vi "PLC.Dial800.vi"(7 "PLC Indicator":refnum<vi>, 8 "Is Child":bool, 9 "Config Dir":path=path "C:/MTE/Circle Test/Config", 10 "Name":string="PLC", 11 "TE Q":refnum<queue>) -> ()   [LabVIEW 2018]
uses:
  SubVIs/PLC.800 Variables.ctl
  <vilib>/KATE/Queues/Q.Element.ctl
  SubVIs/PLC.Dial800.Var URL Item.ctl
  SubVIs/PLC.Dial800.VarNameSelector.ctl
  SubVIs/PLC.Dial800.OPC Server Config.ctl
  SubVIs/PLC.Dial800.VarNames.ctl
  Beckhoff/Dial 750/Controls/PLC750.Connection Config.ctl
  <vilib>/KATE/Queues/Queue Utils.lvlib
  <vilib>/KATE/Scheduler/Scheduler.lvlib
  <vilib>/KATE/Status/Status Utils.lvlib
panel:
  out "Nest":i32
  out "Test State 2":T1(radio)
  out "Connected":bool
  in  "Tab Control":enum32{"Operate", "Config", "Maint"}(tab)
  out "PLC HB Err Msg":string="PLC Hearbeat Error"
  out "PLC HB Err":bool
  in  "SN Set":bool
  in  "SN Input":string caption="SN"
  in  "Reset Clear":bool
  in  "Reset Set":bool
  in  "Run Clear":bool
  in  "Run Set":bool
  in  "Start Clear":bool
  in  "Seq Done FAIL":bool
  in  "Seq Run":bool
  in  "Seq Done PASS":bool
  out "Status":string
  out "SN":string
  out "Test State":T1(radio)
  out "Reading":bool
  out "PLC Variables":T2
  in  "Start Set":bool
  out "Test Running":bool
  out "Result":string
  out "Read Time":timestamp format="%<%.3X>T"
  in  "PLC Read Interval(s)":dbl=0.1 caption="Read Interval(s)" format="%#_13g"
  in  "Read Data":bool
  out "ReadDur(s)":dbl format="%.3f"
  in  "Reset":bool
  out "OPC Server":T3={"IP"="localhost", "Topic"="Stn800", "Server"="RSLinx OPC Server", "VarRoot"="Program:Stn001_90_OffloadMain", "TestPCArray"="TestPC", "VarNames"={"SN"="SN", "Reset"="Reset", "HeartbeatPLC"="HeartbeatPLC", "HeartbeatPC"="HeartbeatTestPC", "Start"="Start", "Running"="Running", "Done"="Done", "Pass"="Pass"}}
  out "Var URLs":T5[](array[typedef])
  in  "PLC HB TimeOut(s)":dbl=5.0 caption="PLC Heartbeat Timeout(s)" format="%#_13g"
  in  "Retry Sec":dbl=2.0 caption="Connect Retry Sec" format="%#_13g"
  out "Error":errorcluster
  in  "Clear Error":bool
  out "Error Time":timestamp format="%<%.3X>T"
  in  "Exit":bool
  in  "Simulate":bool
  in  "Single Step":bool
  in  "Enabled":bool=TRUE
  # "PLC Connection Manager"
  # "Manual Ctrl"
  # "Test Executive Data"
  # "Start"
  # "Running"
  # "Result\nDone"
  # "Simulate TE"
  # "Reset"
  # "(Access path)"
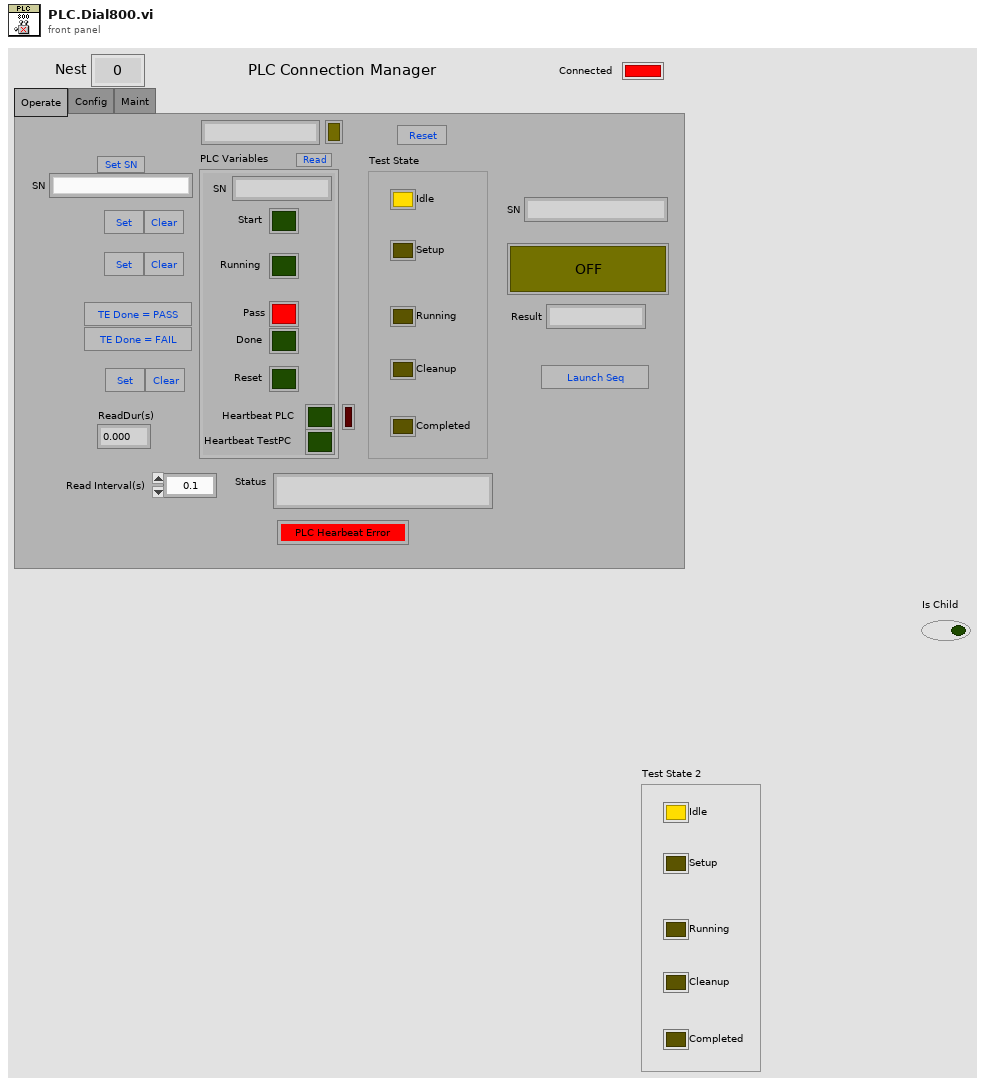
[diagram p1: front panel]
types:
  T1 = enum32{"Idle", "Setup", "Running", "Cleanup", "Completed"}
  T2 = typedef "PLC.800 Variables.ctl" = cluster{"SN":string, "Start":bool, "Pass":bool, "Done":bool, "Running":bool, "Heartbeat PLC":bool, "Heartbeat TestPC":bool, "Reset":bool}
  T3 = typedef "PLC.Dial800.OPC Server Config.ctl" = cluster{"IP":string, "Topic":string, "Server":string, "VarRoot":string, "TestPCArray":string, "VarNames":T4}
  T4 = typedef "PLC.Dial800.VarNames.ctl" = cluster{"SN":string, "Reset":string, "HeartbeatPLC":string, "HeartbeatPC":string, "Start":string, "Running":string, "Done":string, "Pass":string}
  T5 = typedef "PLC.Dial800.Var URL Item.ctl" = cluster{"Var":T6, "URL":string, "Socket ID":refnum<k13>}
  T6 = typedef "PLC.Dial800.VarNameSelector.ctl" = enum16{"SN", "Reset", "HeartBeat_PLC", "Heartbeat_PC", "Start", "Running", "Done", "Pass"}
  T7 = enum32{"invalid app kind", "Development System", "Run Time System", "Student Edition", "Embedded LabVIEW", "Evaluation", "Custom"}
  T8 = enum8{"Enabled", "Disabled", "Disabled and Grayed Out"}
  T9 = enum32{"Invalid", "Standard", "Closed", "Hidden", "Minimized", "Maximized"}
  T10 = typedef "PLC750.Connection Config.ctl" = cluster{"Net ID Target":string, "Net ID Source":string, "IP Address Target":string, "Target Port":u16}
  T11 = cluster{"OPC Server":T3, "Var URLs":T5[], "Data":T2, "Nest":i32, "Connected":bool, "ConCfg":T10, "State":enum32{"Idle", "Setup", "Running", "Cleanup", "Completed"}, "PLC Indicator":refnum<vi>, "HeartBeat":bool, "TE Running":bool, "Cleanup":bool, "Reset":bool, "HB PLC Trans":timestamp, "HB PLC Last State":bool, "PLC HB Err":bool}
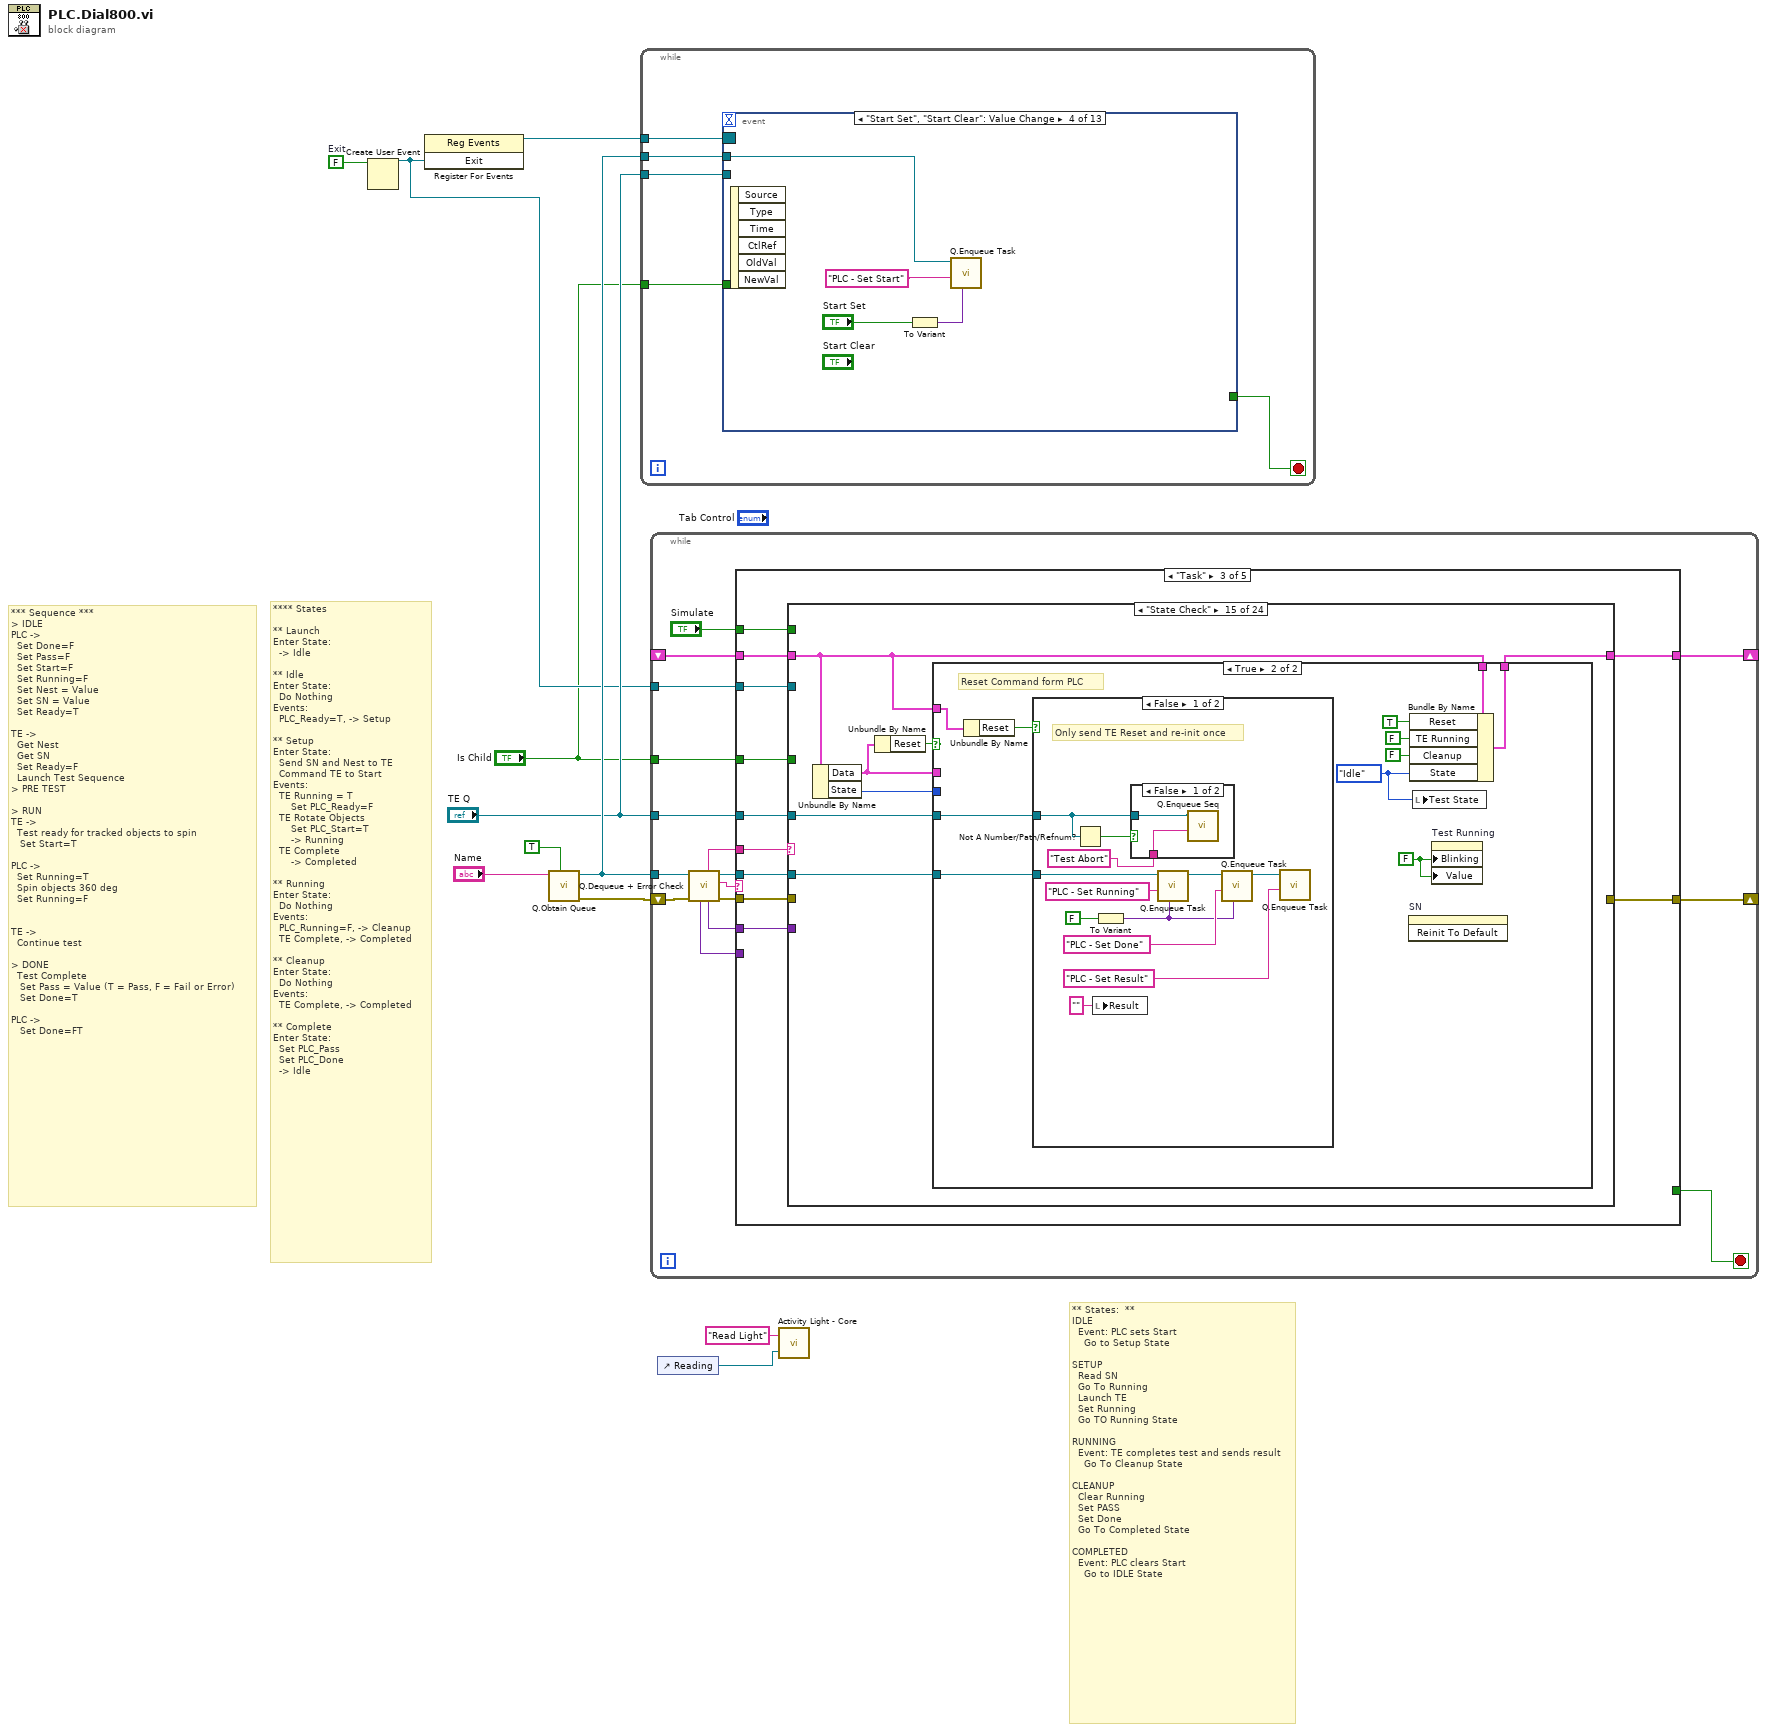
[diagram p0: block diagram]
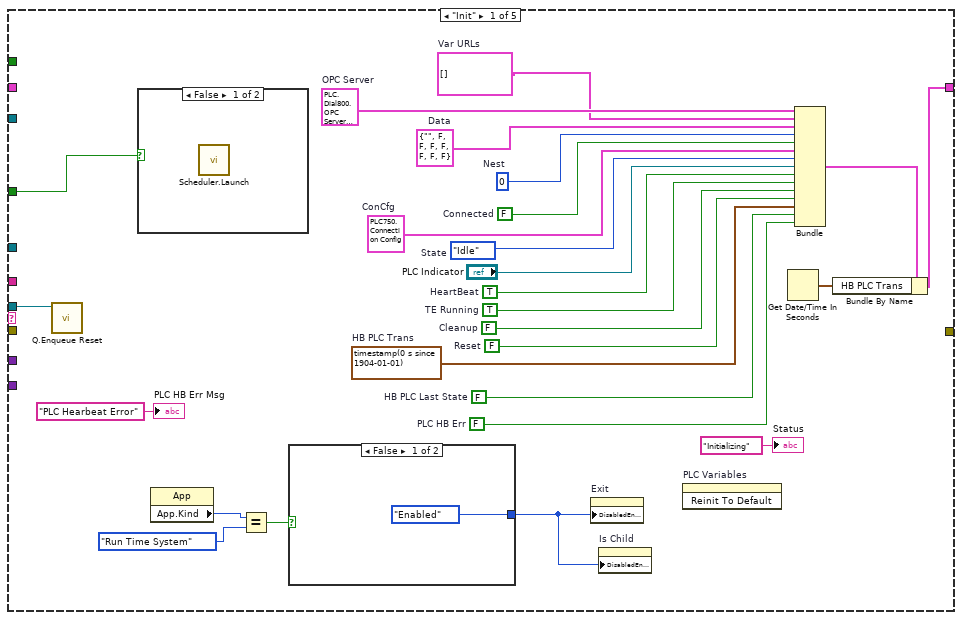
[diagram p2: hidden frame]
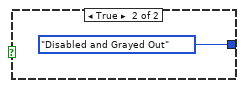
[diagram p3: hidden frame]
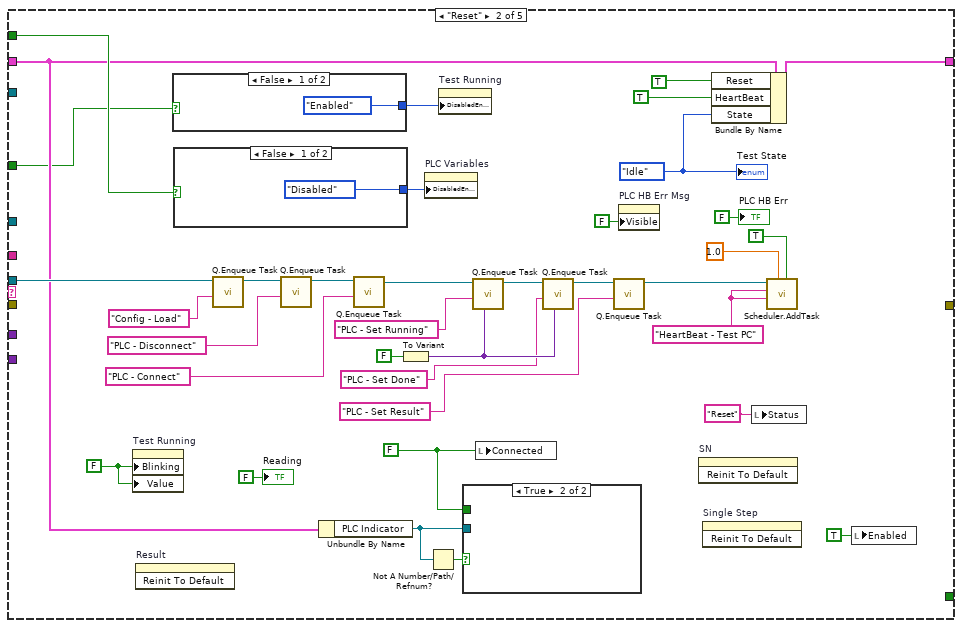
[diagram p5: hidden frame]
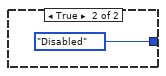
[diagram p6: hidden frame]
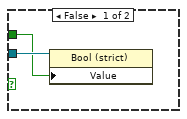
[diagram p7: hidden frame]
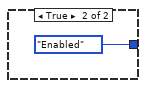
[diagram p8: hidden frame]
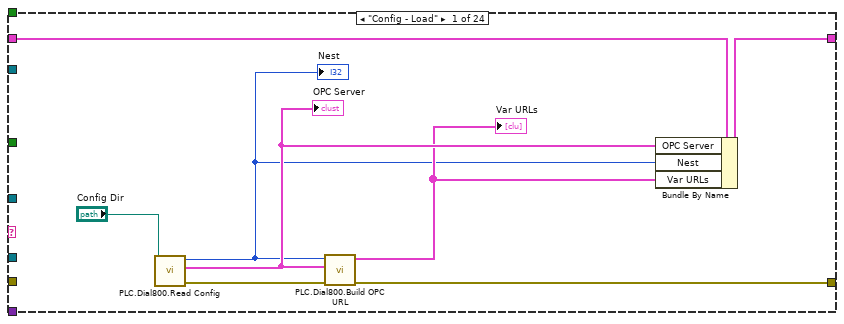
[diagram p9: hidden frame]
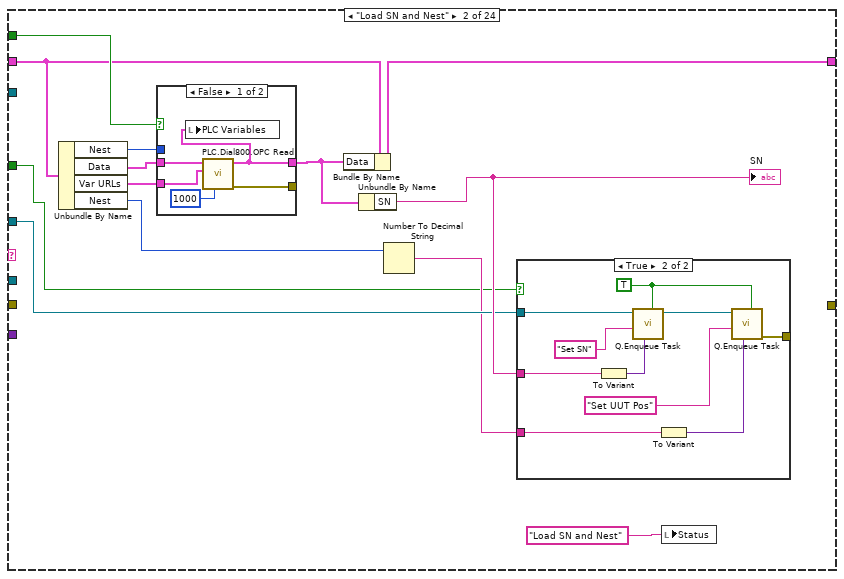
[diagram p10: hidden frame]
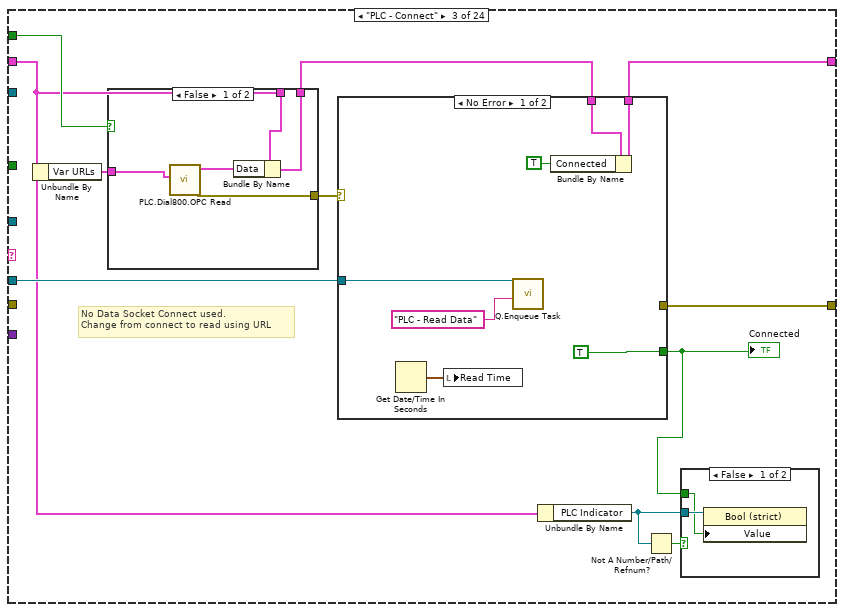
[diagram p13: hidden frame]
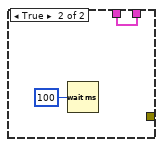
[diagram p15: hidden frame]
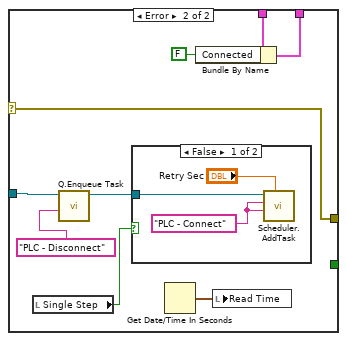
[diagram p16: hidden frame]
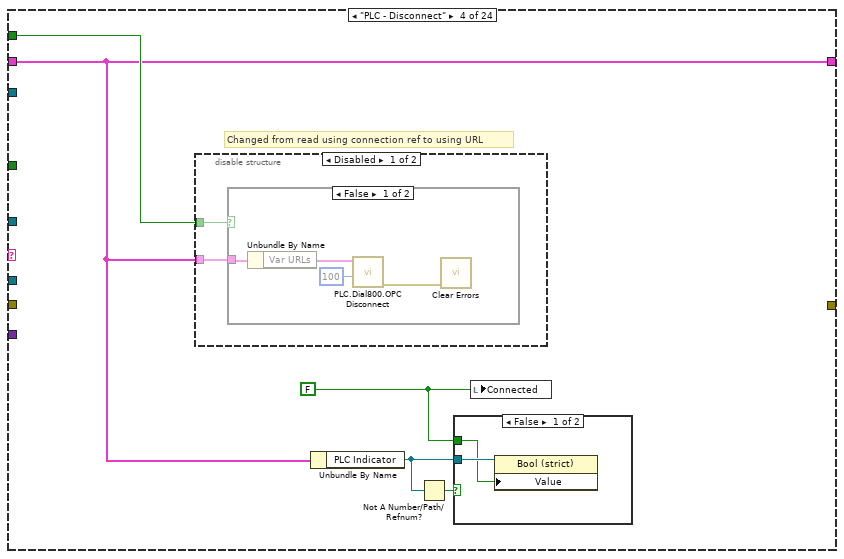
[diagram p18: hidden frame]
diagram:
  w8 = FALSE  # Exit
  # "** States:  ** \nIDLE\n  Event: PLC sets Start\n    Go to Setup State\n\nSETUP\n  Read SN\n  Go To Running\n  Launch TE\n  Set Running\n  Go TO Running State\n\nRUNNING\n  Event: TE completes test and sends result\n    Go To Cleanup State\n\nCLEANUP\n  Clear Running\n  Set PASS\n  Set Done\n  Go To Completed State\n\nCOMPLETED\n  Event: PLC clears Start\n    Go to IDLE State"
  # "**** States\n\n** Launch\nEnter State: \n  -> Idle\n\n** Idle\nEnter State: \n  Do Nothing\nEvents:\n  PLC_Ready=T, -> Setup\n\n** Setup\nEnter State: \n  Send SN and Nest to TE\n  Command TE to Start\nEvents:\n  TE Running = T\n      Set PLC_Ready=F\n  TE Rotate Objects\n      Set PLC_Start=T\n      -> Running\n  TE Complete\n      -> Completed\n\n** Running\nEnter State: \n  Do Nothing\nEvents:\n  PLC_Running=F, -> Cleanup\n  TE Complete, -> Completed\n\n** Cleanup\nEnter State: \n  Do Nothing\nEvents:\n  TE Complete, -> Completed\n\n** Complete\nEnter State: \n  Set PLC_Pass\n  Set PLC_Done \n  -> Idle"
  # "*** Sequence ***\n> IDLE\nPLC -> \n  Set Done=F\n  Set Pass=F\n  Set Start=F\n  Set Running=F\n  Set Nest = Value\n  Set SN = Value\n  Set Ready=T\n\nTE -> \n  Get Nest\n  Get SN\n  Set Ready=F\n  Launch Test Sequence\n> PRE TEST\n  \n> RUN\nTE -> \n  Test ready for tracked objects to spin\n   Set Start=T\n\nPLC -> \n  Set Running=T\n  Spin objects 360 deg\n  Set Running=F\n\n\nTE -> \n  Continue test\n\n> DONE\n  Test Complete\n   Set Pass = Value (T = Pass, F = Fail or Error)\n   Set Done=T\n\nPLC -> \n   Set Done=FT"
  n1 = Create User Event(user event datatype=w8) -> (user event=w4:refnum<user-event>)  [unwired: 1 in, 1 out]
  n2 = register-events(w4) -> (reference out=w7:refnum<event-registration>)  [unwired: 2 in, 1 out]
  n3 = call <vilib>:"Q.Obtain Queue.vi"("Enqueue Init"=TRUE, "Q Name"="Name") -> ("error out"=w5:errorcluster, "Q Out"=w9:refnum<queue>)  [unwired: 7 in, 1 out]
  n4 = while {
    tunnel: w9 -> [w16]
    tunnel: w7 -> [w15]
    tunnel: "TE Q" -> [w14]
    tunnel: "Is Child" -> [w12]
    stop <- w13 stop-if-true
    n5 = event shown="[3] \"Start Set\", \"Start Clear\": Value Change" {
      selector: w15 -> [_ _ _ _ _ _ _ _ _ _ _ _ _]
      dyn-events: _ -> [_ _ _ _ _ _ _ _ _ _ _ _ _]
      timeout: _ -> [_ _ _ _ _ _ _ _ _ _ _ _ _]
      tunnel: w16 -> [_ w17 w18 w23 w27 w31 w33 w39 w45 _ w49 w55 w56]
      tunnel: w14 -> [_ _ _ _ _ _ _ _ _ _ _ _ _]
      tunnel: [_ _ _ _ _ _ _ _ _ TRUE w48 TRUE _] -> w13
      tunnel: w12 -> [_ _ _ _ _ _ _ _ _ _ w47 _ _]
      event "Clear Error": Value Change {
        n6 = event-data() -> ()  [unwired: 1 in, 6 out]
        n7 = invoke on="Error" class="Clust (strict)" method="Reinit To Default"() -> ()  [unwired: 3 in, 3 out]
      }
      event "Reset": Value Change {
        n8 = event-data() -> ()  [unwired: 1 in, 6 out]
        n9 = call <vilib>:"Q.Enqueue Reset.vi"("Q In"=w17) -> ()  [unwired: 9 in, 2 out]
      }
      event "Read Data": Value Change {
        n10 = event-data() -> ()  [unwired: 1 in, 6 out]
        n11 = call <vilib>:"Q.Enqueue Task.vi"("Task Name"="PLC - Read Data", "Q In"=w18) -> ()  [unwired: 8 in, 2 out]
      }
      event "Start Set", "Start Clear": Value Change {
        n12 = event-data() -> ()  [unwired: 1 in, 6 out]
        n13 = To Variant(anything="Start Set") -> (Variant=w21:variant)
        n14 = call <vilib>:"Q.Enqueue Task.vi"("Data1"=w21, "Task Name"="PLC - Set Start", "Q In"=w23) -> ()  [unwired: 7 in, 2 out]
      }
      event "Run Set", "Run Clear": Value Change {
        n15 = event-data() -> ()  [unwired: 1 in, 6 out]
        n16 = To Variant(anything="Run Set") -> (Variant=w25:variant)
        n17 = call <vilib>:"Q.Enqueue Task.vi"("Data1"=w25, "Task Name"="PLC - Set Running", "Q In"=w27) -> ()  [unwired: 7 in, 2 out]
      }
      event "Reset Set", "Reset Clear": Value Change {
        n18 = event-data() -> ()  [unwired: 1 in, 6 out]
        n19 = To Variant(anything="Reset Set") -> (Variant=w29:variant)
        n20 = call <vilib>:"Q.Enqueue Task.vi"("Data1"=w29, "Task Name"="PLC - Set Reset", "Q In"=w31) -> ()  [unwired: 7 in, 2 out]
      }
      event "SN Set": Value Change {
        n21 = event-data() -> ()  [unwired: 1 in, 6 out]
        n22 = call <vilib>:"Q.Enqueue Task.vi"("Task Name"="PLC - Set SN", "Q In"=w33) -> ()  [unwired: 8 in, 2 out]
      }
      event "Seq Done PASS": Value Change {
        n23 = event-data() -> ()  [unwired: 1 in, 6 out]
        n24 = To Variant(anything="PASS") -> (Variant=w34:variant)
        n25 = call <vilib>:"Q.Enqueue Task.vi"("Data1"=w34, "Task Name"="TE Result", "Q In"=w39) -> ("Q Out"=w37:refnum<queue>)  [unwired: 7 in, 1 out]
        n26 = call <vilib>:"Q.Enqueue Task.vi"("Task Name"="TE Complete", "Q In"=w37) -> ()  [unwired: 8 in, 2 out]
      }
      event "Seq Done FAIL": Value Change {
        n27 = event-data() -> ()  [unwired: 1 in, 6 out]
        n28 = To Variant(anything="FAIL") -> (Variant=w40:variant)
        n29 = call <vilib>:"Q.Enqueue Task.vi"("Data1"=w40, "Task Name"="TE Result", "Q In"=w45) -> ("Q Out"=w43:refnum<queue>)  [unwired: 7 in, 1 out]
        n30 = call <vilib>:"Q.Enqueue Task.vi"("Task Name"="TE Complete", "Q In"=w43) -> ()  [unwired: 8 in, 2 out]
      }
      event User Event {
        n31 = event-data() -> ()  [unwired: 1 in, 4 out]
      }
      event Panel Close? {
        n32 = event-data() -> ()  [unwired: 1 in, 4 out]
        n33 = case shown="False" w47 {
          tunnel: w49 -> [w52 _]
          tunnel: [TRUE _] -> w48
          frame False {
            n34 = call <vilib>:"Q.Enqueue Exit.vi"("Q In"=w52) -> ()  [unwired: 9 in, 2 out]
          }
          frame True {
            n35 = control-ref of="This VI"() -> (w53:refnum<vi>)
            n36 = invoke class="VI" method="FP.Close"(reference=w53) -> ()  [unwired: 2 in, 3 out]
          }
        }
        n37 = event-data("Discard?"=TRUE) -> ()  [unwired: 1 in, 1 out]
      }
      event "Exit": Value Change {
        n38 = event-data() -> ()  [unwired: 1 in, 6 out]
        n39 = call <vilib>:"Q.Enqueue Exit.vi"("Q In"=w55) -> ()  [unwired: 9 in, 2 out]
      }
      event "Seq Run": Value Change {
        n40 = event-data() -> ()  [unwired: 1 in, 6 out]
        n41 = call <vilib>:"Q.Enqueue Task.vi"("Task Name"="TE Running", "Q In"=w56) -> ()  [unwired: 8 in, 2 out]
      }
    }
  }
  n42 = while {
    tunnel: w9 -> [w73]
    shift-right: [w65] -> _
    shift-left: _ -> [w72]
    tunnel: "TE Q" -> [w63]
    shift-right: [w61] -> _
    shift-left: w5 -> [w62]
    tunnel: w4 -> [w60]
    tunnel: "Is Child" -> [w58]
    stop <- w64 stop-if-true
    n43 = call <vilib>:"Q.Dequeue + Error Check.vi"("Error In"=w62, "Q In"=w73) -> ("error out"=w69:errorcluster, "Cmd"=w71:string, "Q Out"=w70:refnum<queue>, "Data1"=w67:variant, "Sub"=w68:string, "Data2"=w66:variant)  [unwired: 4 in]
    n44 = case shown="\"Task\"" w71 {
      tunnel: w72 -> [_ w122 w150 w715 w726]
      tunnel: w70 -> [w96 w132 w152 _ w725]
      tunnel: w69 -> [_ _ w151 w718 _]
      tunnel: w68 -> [_ _ w154 w719 _]
      tunnel: w67 -> [_ _ w153 w716 _]
      tunnel: w66 -> [_ _ _ _ _]
      tunnel: [w75 w133 w149 w715 w726] -> w65
      tunnel: [_ _ _ _ TRUE] -> w64
      tunnel: w63 -> [_ _ w145 _ _]
      tunnel: [_ _ w148 _ _] -> w61
      tunnel: w60 -> [_ _ w147 _ w733]
      tunnel: "Simulate" -> [_ w128 w146 _ w727]
      tunnel: w58 -> [w92 w120 w144 _ w731]
      frame "Init" {
        w77 = FALSE  # PLC HB Err
        w79 = FALSE  # HB PLC Last State
        w80 = timestamp(0 s since 1904-01-01)  # HB PLC Trans
        w81 = FALSE  # Reset
        w82 = FALSE  # Cleanup
        w83 = TRUE  # TE Running
        w84 = TRUE  # HeartBeat
        w85 = T2 {"SN"="", "Start"=FALSE, "Pass"=FALSE, "Done"=FALSE, "Running"=FALSE, "Heartbeat PLC"=FALSE, "Heartbeat TestPC"=FALSE, "Reset"=FALSE}  # Data
        w86 = T5[] []  # Var URLs
        w87 = T3 {"IP"="localhost", "Topic"="Stn800", "Server"="RSLinx OPC Server", "VarRoot"="Program:Stn001_90_OffloadMain", "TestPCArray"="TestPC", "VarNames"={"SN"="SN", "Reset"="Reset", "HeartbeatPLC"="HeartbeatPLC", "HeartbeatPC"="HeartbeatTestPC", "Start"="Start", "Running"="Running", "Done"="Done", "Pass"="Pass"}}  # OPC Server
        w95 = T1."Idle"  # State
        w97 = T10 {"Net ID Target"="5.49.203.74.1.1", "Net ID Source"="192.168.1.18.1.1", "IP Address Target"="172.16.113.5", "Target Port"=851}  # ConCfg
        w98 = FALSE  # Connected
        w99 = 0  # Nest
        n45 = call <vilib>:"Q.Enqueue Reset.vi"("Q In"=w96) -> ()  [unwired: 9 in, 2 out]
        n46 = case shown="False" w92 {
          frame False {
            n47 = call <vilib>:"Scheduler.Launch.vi"() -> ()  [unwired: 9 in, 3 out]
          }
          frame True {
          }
        }
        n48 = property class="App"() -> ("App.Kind"=w90:T7)  [unwired: 2 in, 2 out]
        n49 = Equal?(x=w90, y=T7."Run Time System" ("Application:Kind")) -> (x = y?=w88:bool)
        n50 = case shown="False" w88 {
          tunnel: [T8."Enabled" ("Disabled") T8."Disabled and Grayed Out" ("Disabled")] -> w91
          frame False {
          }
          frame True {
          }
        }
        n51 = property on="Exit" class="Bool"("DisabledEnum"=w91) -> ()  [unwired: 2 in, 2 out]
        n52 = property on="Is Child" class="Bool (strict)"("DisabledEnum"=w91) -> ()  [unwired: 2 in, 2 out]
        n53 = invoke on="PLC Variables" class="Clust (strict)" method="Reinit To Default"() -> ()  [unwired: 3 in, 3 out]
        n54 = Get Date/Time In Seconds() -> (seconds since 1Jan1904=w74:timestamp)
        n55 = Bundle("OPC Server"=w87, "Var URLs"=w86, "Data"=w85, "Nest"=w99, "Connected"=w98, "ConCfg"=w97, "State"=w95, "PLC Indicator"="PLC Indicator", "HeartBeat"=w84, "TE Running"=w83, "Cleanup"=w82, "Reset"=w81, "HB PLC Trans"=w80, "HB PLC Last State"=w79, "PLC HB Err"=w77) -> (w76:T11)  [unwired: 1 in]
        n56 = Bundle By Name(cluster=w76, "HB PLC Trans"=w74) -> (w75:T11)
        "Status" <- "Initializing" ("Activity")
        "PLC HB Err Msg" <- "PLC Hearbeat Error" ("PLC HB Err Msg")
      }
      frame "Reset" {
        w117 = "HeartBeat - Test PC" ("Sched Name")
        w129 = T1."Idle" ("Test State")
        w123 = FALSE ("Connected")
        w131 = FALSE ("Blinking")
        n57 = property on="Test Running" class="Bool (strict)"("Blinking"=w131, "Value"=w131) -> ()  [unwired: 2 in, 2 out]
        n58 = invoke on="Result" class="Str" method="Reinit To Default"() -> ()  [unwired: 3 in, 3 out]
        n59 = case shown="False" w120 {
          tunnel: [T8."Enabled" ("Disabled") T8."Disabled" ("Disabled")] -> w121
          frame False {
          }
          frame True {
          }
        }
        n60 = case shown="False" w128 {
          tunnel: [T8."Disabled" ("Disabled") T8."Enabled" ("Disabled")] -> w127
          frame False {
          }
          frame True {
          }
        }
        n61 = call <vilib>:"Q.Enqueue Task.vi"("Task Name"="Config - Load", "Q In"=w132) -> ("Q Out"=w134:refnum<queue>)  [unwired: 8 in, 1 out]
        n62 = call <vilib>:"Q.Enqueue Task.vi"("Task Name"="PLC - Disconnect", "Q In"=w134) -> ("Q Out"=w113:refnum<queue>)  [unwired: 8 in, 1 out]
        n63 = Unbundle By Name(w122) -> ("PLC Indicator"=w124:refnum<vi>)
        n64 = call <vilib>:"Q.Enqueue Task.vi"("Task Name"="PLC - Connect", "Q In"=w113) -> ("Q Out"=w105:refnum<queue>)  [unwired: 8 in, 1 out]
        n65 = To Variant(anything=FALSE) -> (Variant=w111:variant)
        n66 = property on="PLC Variables" class="Clust (strict)"("DisabledEnum"=w127) -> ()  [unwired: 2 in, 2 out]
        n67 = Not A Number/Path/Refnum?(number/path/refnum=w124) -> (NaN/Path/Refnum?=w125:bool)
        n68 = property on="Test Running" class="Bool (strict)"("DisabledEnum"=w121) -> ()  [unwired: 2 in, 2 out]
        n69 = case shown="True" w125 {
          tunnel: w124 -> [w141 _]
          tunnel: w123 -> [w140 _]
          frame False {
            n70 = property class="Bool (strict)"(reference=w141, "Value"=w140) -> ()  [unwired: 1 in, 2 out]
          }
          frame True {
          }
        }
        n71 = call <vilib>:"Q.Enqueue Task.vi"("Data1"=w111, "Task Name"="PLC - Set Running", "Q In"=w105) -> ("Q Out"=w110:refnum<queue>)  [unwired: 7 in, 1 out]
        n72 = local write "Connected"(w123) -> ()
        n73 = call <vilib>:"Q.Enqueue Task.vi"("Data1"=w111, "Task Name"="PLC - Set Done", "Q In"=w110) -> ("Q Out"=w112:refnum<queue>)  [unwired: 7 in, 1 out]
        n74 = call <vilib>:"Q.Enqueue Task.vi"("Task Name"="PLC - Set Result", "Q In"=w112) -> ("Q Out"=w104:refnum<queue>)  [unwired: 8 in, 1 out]
        n75 = property on="PLC HB Err Msg" class="Str"("Visible"=FALSE) -> ()  [unwired: 2 in, 2 out]
        n76 = invoke on="SN" class="Str" method="Reinit To Default"() -> ()  [unwired: 3 in, 3 out]
        n77 = invoke on="Single Step" class="Bool (strict)" method="Reinit To Default"() -> ()  [unwired: 3 in, 3 out]
        n78 = Bundle By Name(cluster=w122, "Reset"=TRUE ("HeartBeat"), "HeartBeat"=TRUE, "State"=w129) -> (w133:T11)
        n79 = local write "Status"("Reset" ("Activity")) -> ()
        n80 = call <vilib>:"Scheduler.AddTask.vi"("Recurring"=TRUE, "Interval(s)"=1.0, "Task Name"=w117, "Sched Name"=w117, "Q In"=w104) -> ()  [unwired: 5 in, 2 out]
        n81 = local write "Enabled"(TRUE ("Enabled")) -> ()
        "Reading" <- FALSE ("Reading")
        "Test State" <- w129
        "PLC HB Err" <- FALSE ("PLC HB Err")
      }
      frame "Task" {
        n82 = case shown="\"State Check\"" w154 {
          tunnel: w153 -> [_ _ _ _ _ w284 w311 w338 w365 _ _ _ _ _ _ _ _ w667 _ _ _ w703 _ _]
          tunnel: w152 -> [_ _ w200 _ w256 _ _ _ _ _ _ w443 w473 w502 w532 _ w660 _ _ w671 w674 w700 w710 _]
          tunnel: w151 -> [_ _ _ _ w244 _ _ _ _ _ _ _ _ _ _ _ _ _ _ _ _ _ _ _]
          tunnel: w150 -> [w160 w164 w193 w232 w255 w281 w308 w335 w362 w390 w419 w446 w479 w500 w528 w652 w663 w668 w669 w670 w677 w698 w705 w713]
          tunnel: [w161 w167 w201 w232 w254 w281 w308 w335 w362 w390 w419 w449 w478 w499 w531 w652 w662 w668 w669 w670 w676 w697 w704 w713] -> w149
          tunnel: [w157 _ w199 _ w251 w287 w314 w341 w368 w393 w423 w451 _ _ _ _ _ _ _ _ _ _ _ _] -> w148
          tunnel: w147 -> [_ _ _ _ _ _ _ _ _ _ _ _ _ _ _ _ _ _ _ _ _ _ _ _]
          tunnel: w146 -> [_ w165 w197 w235 w249 w285 w312 w339 w366 w391 w420 w453 _ _ _ _ _ _ _ _ w673 _ _ _]
          tunnel: w145 -> [_ w173 _ _ _ _ _ _ _ _ _ _ _ w503 w530 _ _ _ _ _ w679 _ _ _]
          tunnel: w144 -> [_ w171 _ _ _ _ _ _ _ _ _ _ _ _ _ _ _ _ _ _ w678 _ _ _]
          frame "Config - Load" {
            n83 = call "PLC.Dial800.Read Config.vi"("Config Folder"="Config Dir") -> ("error out"=w158:errorcluster, "OPC Server"=w159:T3, "Nest"=w155:i32)  [unwired: 8 in]
            "OPC Server" <- w159
            "Nest" <- w155
            n84 = call "PLC.Dial800.Build OPC URL.vi"("error in (no error)"=w158, "OPC Server"=w159, "Nest"=w155) -> ("error out"=w157:errorcluster, "Var URLs"=w156:T5[])  [unwired: 7 in]
            "Var URLs" <- w156
            n85 = Bundle By Name(cluster=w160, "OPC Server"=w159, "Nest"=w155, "Var URLs"=w156) -> (w161:T11)
          }
          frame "Load SN and Nest" {
            n86 = Unbundle By Name(w164) -> ("Nest"=w168:i32, "Data"=w169:T2, "Var URLs"=w170:T5[], "Nest"=w163:i32)
            n87 = case shown="False" w165 {
              tunnel: w168 -> [_ _]
              tunnel: w169 -> [w180 w181]
              tunnel: w170 -> [w179 _]
              tunnel: [w176 w181] -> w166
              tunnel: [w178 _] -> _
              frame False {
                n88 = call "PLC.Dial800.OPC Read.vi"("Timeout_ms"=1000, "Var URLs"=w179, "PLC Variables In"=w180) -> ("error out"=w178:errorcluster, "PLC Variables"=w176:T2)  [unwired: 6 in, 1 out]
                n89 = local write "PLC Variables"(w176) -> ()
              }
              frame True {
              }
            }
            n90 = Bundle By Name(cluster=w164, "Data"=w166) -> (w167:T11)
            n91 = Unbundle By Name(w166) -> ("SN"=w174:string)
            "SN" <- w174
            n92 = Number To Decimal String(number=w163) -> (decimal integer string=w172:string)  [unwired: 1 in]
            n93 = case shown="True" w171 {
              tunnel: w174 -> [_ w191]
              tunnel: w173 -> [_ w190]
              tunnel: w172 -> [_ w189]
              tunnel: [_ w183] -> _
              frame False {
              }
              frame True {
                w182 = TRUE ("Top of Q")
                n94 = To Variant(anything=w191) -> (Variant=w188:variant)
                n95 = call <vilib>:"Q.Enqueue Task.vi"("Top of Q"=w182, "Data1"=w188, "Task Name"="Set SN", "Q In"=w190) -> ("Q Out"=w184:refnum<queue>)  [unwired: 6 in, 1 out]
                n96 = To Variant(anything=w189) -> (Variant=w186:variant)
                n97 = call <vilib>:"Q.Enqueue Task.vi"("Top of Q"=w182, "Data1"=w186, "Task Name"="Set UUT Pos", "Q In"=w184) -> ("error out"=w183:errorcluster)  [unwired: 6 in, 1 out]
              }
            }
            n98 = local write "Status"("Load SN and Nest" ("Activity")) -> ()
          }
          frame "PLC - Connect" {
            # "No Data Socket Connect used.\nChange from connect to read using URL"
            n99 = Unbundle By Name(w193) -> ("Var URLs"=w198:T5[])
            n100 = case shown="False" w197 {
              tunnel: [w205 _] -> w202
              tunnel: w198 -> [w207 _]
              tunnel: w193 -> [w209 w210]
              tunnel: [w208 w210] -> w192
              frame False {
                n101 = call "PLC.Dial800.OPC Read.vi"("Var URLs"=w207) -> ("error out"=w205:errorcluster, "PLC Variables"=w206:T2)  [unwired: 8 in, 1 out]
                n102 = Bundle By Name(cluster=w209, "Data"=w206) -> (w208:T11)
              }
              frame True {
                n103 = Wait (ms)(milliseconds to wait=u32 100) -> ()  [unwired: 1 out]
              }
            }
            n104 = case shown="No Error" w202 {
              selector: w202 -> [_ w224]
              tunnel: [w218 w226] -> w201
              tunnel: w192 -> [w217 w227]
              tunnel: w200 -> [w214 w221]
              tunnel: [TRUE _] -> w194
              tunnel: [_ w224] -> w199
              frame No Error {
                n105 = Get Date/Time In Seconds() -> (seconds since 1Jan1904=w212:timestamp)
                n106 = local write "Read Time"(w212) -> ()
                n107 = call <vilib>:"Q.Enqueue Task.vi"("Task Name"="PLC - Read Data" ("Sched Name"), "Q In"=w214) -> ()  [unwired: 8 in, 2 out]
                n108 = Bundle By Name(cluster=w217, "Connected"=TRUE) -> (w218:T11)
              }
              frame Error {
                n109 = local read "Single Step"() -> (w223:bool)
                n110 = call <vilib>:"Q.Enqueue Task.vi"("Task Name"="PLC - Disconnect" ("Sched Name"), "Q In"=w221) -> ("Q Out"=w220:refnum<queue>)  [unwired: 8 in, 1 out]
                n111 = case shown="False" w223 {
                  tunnel: w220 -> [w228 _]
                  frame False {
                    w230 = "PLC - Connect" ("Sched Name")
                    n112 = call <vilib>:"Scheduler.AddTask.vi"("Interval(s)"="Retry Sec", "Task Name"=w230, "Sched Name"=w230, "Q In"=w228) -> ()  [unwired: 6 in, 2 out]
                  }
                  frame True {
                  }
                }
                n113 = Get Date/Time In Seconds() -> (seconds since 1Jan1904=w222:timestamp)
                n114 = Bundle By Name(cluster=w227, "Connected"=FALSE) -> (w226:T11)
                n115 = local write "Read Time"(w222) -> ()
              }
            }
            "Connected" <- w194
            n116 = Unbundle By Name(w193) -> ("PLC Indicator"=w195:refnum<vi>)
            n117 = Not A Number/Path/Refnum?(number/path/refnum=w195) -> (NaN/Path/Refnum?=w196:bool)
            n118 = case shown="False" w196 {
              tunnel: w195 -> [w204 _]
              tunnel: w194 -> [w203 _]
              frame False {
                n119 = property class="Bool (strict)"(reference=w204, "Value"=w203) -> ()  [unwired: 1 in, 2 out]
              }
              frame True {
              }
            }
          }
          frame "PLC - Disconnect" {
            w231 = FALSE ("Connected")
            # "Changed from read using connection ref to using URL"
            n120 = disable-structure shown="Disabled" {
              disable-tunnel: w235 -> [w237 _]
              disable-tunnel: w232 -> [w236 _]
              frame Disabled {
                n121 = case shown="False" w237 {
                  tunnel: w236 -> [w241 _]
                  frame False {
                    n122 = Unbundle By Name(w241) -> ("Var URLs"=w240:T5[])
                    n123 = call "PLC.Dial800.OPC Disconnect.vi"("ms timeout (1000)"=100, "Var URLs In"=w240) -> ("error out"=w238:errorcluster)  [unwired: 9 in]
                    n124 = call <vilib>:"Clear Errors.vi"("error in (no error)"=w238) -> ()  [unwired: 5 in, 2 out]
                  }
                  frame True {
                  }
                }
              }
              frame Enabled {
              }
            }
            n125 = Unbundle By Name(w232) -> ("PLC Indicator"=w233:refnum<vi>)
            n126 = Not A Number/Path/Refnum?(number/path/refnum=w233) -> (NaN/Path/Refnum?=w234:bool)
            n127 = case shown="False" w234 {
              tunnel: w233 -> [w243 _]
              tunnel: w231 -> [w242 _]
              frame False {
                n128 = property class="Bool (strict)"(reference=w243, "Value"=w242) -> ()  [unwired: 1 in, 2 out]
              }
              frame True {
              }
            }
            n129 = local write "Connected"(w231) -> ()
          }
          frame "PLC - Read Data" {
            n130 = Unbundle By Name(w255) -> ("Data"=w246:T2, "Var URLs"=w253:T5[])
            n131 = Get Date/Time In Seconds() -> (seconds since 1Jan1904=→"Read Time":timestamp)
            n132 = local write "Status"("Read" ("Activity")) -> ()
            n133 = case shown="False" w249 {
              tunnel: w253 -> [w260 _]
              tunnel: [w264 _] -> w252
              tunnel: w244 -> [w263 _]
              tunnel: [w262 w265] -> w247
              tunnel: w246 -> [w261 _]
              frame False {
                n134 = call "PLC.Dial800.OPC Read.vi"("Timeout_ms"=500, "Waif for Update"=FALSE, "error in (no error)"=w263, "Var URLs"=w260, "PLC Variables In"=w261) -> ("error out"=w264:errorcluster, "Duration(s)"=→"ReadDur(s)":dbl, "PLC Variables"=w262:T2)  [unwired: 4 in]
                "PLC Variables" <- w262
              }
              frame True {
                n135 = local read "PLC Variables"() -> (w265:T2)
                n136 = Wait (ms)(milliseconds to wait=u32 100) -> ()  [unwired: 1 out]
              }
            }
            n137 = call <vilib>:"Activity Light - Pulse.vi"("Name"="Read Light" ("Q Name")) -> ()  [unwired: 10 in, 1 out]
            n138 = Bundle By Name(cluster=w255, "Data"=w247) -> (w254:T11)
            n139 = case shown="No Error" w252 {
              selector: w252 -> [_ w278]
              tunnel: w256 -> [w269 w275]
              tunnel: [_ w278] -> w251
              frame No Error {
                n140 = call <vilib>:"Q.Enqueue Task.vi"("Task Name"="State Check", "Q In"=w269) -> ("Q Out"=w268:refnum<queue>)  [unwired: 8 in, 1 out]
                n141 = case shown="False" "Single Step" {
                  tunnel: w268 -> [w272 _]
                  frame False {
                    w273 = "PLC - Read Data" ("Sched Name")
                    n142 = call <vilib>:"Scheduler.AddTask.vi"("Interval(s)"="PLC Read Interval(s)", "Task Name"=w273, "Sched Name"=w273, "Q In"=w272) -> ()  [unwired: 6 in, 2 out]
                  }
                  frame True {
                  }
                }
              }
              frame Error {
                w279 = "PLC - Connect" ("Sched Name")
                n143 = call <vilib>:"Q.Enqueue Task.vi"("Task Name"="PLC - Disconnect" ("Sched Name"), "Q In"=w275) -> ("Q Out"=w274:refnum<queue>)  [unwired: 8 in, 1 out]
                n144 = local read "Retry Sec"() -> (w277:dbl)
                n145 = call <vilib>:"Scheduler.AddTask.vi"("Interval(s)"=w277, "Task Name"=w279, "Sched Name"=w279, "Q In"=w274) -> ()  [unwired: 6 in, 2 out]
              }
            }
          }
          frame "PLC - Set Done" {
            n146 = Variant To Data(type=FALSE, Variant=w284) -> (data=w282:bool)  [unwired: 1 in, 1 out]
            n147 = Unbundle By Name(w281) -> ("Connected"=w280:bool)
            n148 = case shown="True" w280 {
              tunnel: [_ w291] -> w287
              tunnel: w281 -> [_ w290]
              tunnel: w285 -> [_ w289]
              tunnel: w282 -> [_ w288]
              frame False {
              }
              frame True {
                n149 = case shown="False" w289 {
                  tunnel: [w294 _] -> w291
                  tunnel: w290 -> [w297 _]
                  tunnel: w288 -> [w293 w303]
                  frame False {
                    n150 = Unbundle By Name(w297) -> ("Var URLs"=w296:T5[])
                    n151 = for {
                      tunnel: w296 -> [w302] mode=indexing
                      tunnel: [w298] -> w295
                      stop <- w299 stop-if-true
                      n152 = Unbundle By Name(w302) -> ("URL"=w298:string, "Var"=w301:T6)
                      n153 = Equal?(x=w301, y=PLC.Dial800.VarNameSelector."Done" ("Var")) -> (x = y?=w299:bool)
                    }
                    n154 = DataSocket Write(9:100 ("ms timeout (0)"), 10:w293, 11:w295) -> (0:w294:errorcluster)  [unwired: 1 in, 2 out]
                  }
                  frame True {
                    n155 = local read "PLC Variables"() -> (w305:T2)
                    n156 = Bundle By Name(cluster=w305, "Done"=w303) -> (w306:T2)
                    n157 = Wait (ms)(milliseconds to wait=u32 100) -> ()  [unwired: 1 out]
                    n158 = local write "PLC Variables"(w306) -> ()
                  }
                }
              }
            }
            n159 = local write "Status"("Set Done" ("Activity")) -> ()
          }
          frame "PLC - Set Start" {
            n160 = Variant To Data(type=FALSE, Variant=w311) -> (data=w309:bool)  [unwired: 1 in, 1 out]
            n161 = Unbundle By Name(w308) -> ("Connected"=w307:bool)
            n162 = case shown="True" w307 {
              tunnel: [_ w318] -> w314
              tunnel: w308 -> [_ w317]
              tunnel: w312 -> [_ w316]
              tunnel: w309 -> [_ w315]
              frame False {
              }
              frame True {
                n163 = case shown="False" w316 {
                  tunnel: [w321 _] -> w318
                  tunnel: w317 -> [w324 _]
                  tunnel: w315 -> [w320 w330]
                  frame False {
                    n164 = Unbundle By Name(w324) -> ("Var URLs"=w323:T5[])
                    n165 = for {
                      tunnel: w323 -> [w329] mode=indexing
                      tunnel: [w325] -> w322
                      stop <- w326 stop-if-true
                      n166 = Unbundle By Name(w329) -> ("URL"=w325:string, "Var"=w328:T6)
                      n167 = Equal?(x=w328, y=PLC.Dial800.VarNameSelector."Start" ("Var")) -> (x = y?=w326:bool)
                    }
                    n168 = DataSocket Write(9:100 ("ms timeout (0)"), 10:w320, 11:w322) -> (0:w321:errorcluster)  [unwired: 1 in, 2 out]
                  }
                  frame True {
                    n169 = local read "PLC Variables"() -> (w332:T2)
                    n170 = Bundle By Name(cluster=w332, "Start"=w330) -> (w333:T2)
                    n171 = Wait (ms)(milliseconds to wait=u32 100) -> ()  [unwired: 1 out]
                    n172 = local write "PLC Variables"(w333) -> ()
                  }
                }
              }
            }
            n173 = local write "Status"("Set Start" ("Activity")) -> ()
          }
          frame "PLC - Set Running" {
            n174 = Variant To Data(type=FALSE, Variant=w338) -> (data=w336:bool)  [unwired: 1 in, 1 out]
            n175 = Unbundle By Name(w335) -> ("Connected"=w334:bool)
            n176 = case shown="True" w334 {
              tunnel: [_ w345] -> w341
              tunnel: w335 -> [_ w344]
              tunnel: w339 -> [_ w343]
              tunnel: w336 -> [_ w342]
              frame False {
              }
              frame True {
                n177 = case shown="False" w343 {
                  tunnel: [w348 _] -> w345
                  tunnel: w344 -> [w351 _]
                  tunnel: w342 -> [w347 w357]
                  frame False {
                    n178 = Unbundle By Name(w351) -> ("Var URLs"=w350:T5[])
                    n179 = for {
                      tunnel: w350 -> [w356] mode=indexing
                      tunnel: [w352] -> w349
                      stop <- w353 stop-if-true
                      n180 = Unbundle By Name(w356) -> ("URL"=w352:string, "Var"=w355:T6)
                      n181 = Equal?(x=w355, y=PLC.Dial800.VarNameSelector."Running" ("Var")) -> (x = y?=w353:bool)
                    }
                    n182 = DataSocket Write(9:100 ("ms timeout (0)"), 10:w347, 11:w349) -> (0:w348:errorcluster)  [unwired: 1 in, 2 out]
                  }
                  frame True {
                    n183 = local read "PLC Variables"() -> (w359:T2)
                    n184 = Bundle By Name(cluster=w359, "Running"=w357) -> (w360:T2)
                    n185 = Wait (ms)(milliseconds to wait=u32 100) -> ()  [unwired: 1 out]
                    n186 = local write "PLC Variables"(w360) -> ()
                  }
                }
              }
            }
            n187 = local write "Status"("Set Running" ("Activity")) -> ()
          }
          frame "PLC - Set Reset" {
            n188 = Variant To Data(type=FALSE, Variant=w365) -> (data=w363:bool)  [unwired: 1 in, 1 out]
            n189 = Unbundle By Name(w362) -> ("Connected"=w361:bool)
            n190 = case shown="True" w361 {
              tunnel: [_ w372] -> w368
              tunnel: w362 -> [_ w371]
              tunnel: w366 -> [_ w370]
              tunnel: w363 -> [_ w369]
              frame False {
              }
              frame True {
                n191 = case shown="False" w370 {
                  tunnel: [w375 _] -> w372
                  tunnel: w371 -> [w378 _]
                  tunnel: w369 -> [w374 w384]
                  frame False {
                    n192 = Unbundle By Name(w378) -> ("Var URLs"=w377:T5[])
                    n193 = for {
                      tunnel: w377 -> [w383] mode=indexing
                      tunnel: [w379] -> w376
                      stop <- w380 stop-if-true
                      n194 = Unbundle By Name(w383) -> ("URL"=w379:string, "Var"=w382:T6)
                      n195 = Equal?(x=w382, y=PLC.Dial800.VarNameSelector."Reset" ("Var")) -> (x = y?=w380:bool)
                    }
                    n196 = DataSocket Write(9:100 ("ms timeout (0)"), 10:w374, 11:w376) -> (0:w375:errorcluster)  [unwired: 1 in, 2 out]
                  }
                  frame True {
                    n197 = local read "PLC Variables"() -> (w386:T2)
                    n198 = Bundle By Name(cluster=w386, "Reset"=w384) -> (w387:T2)
                    n199 = Wait (ms)(milliseconds to wait=u32 100) -> ()  [unwired: 1 out]
                    n200 = local write "PLC Variables"(w387) -> ()
                  }
                }
              }
            }
            n201 = local write "Status"("Set Reset" ("Activity")) -> ()
          }
          frame "PLC - Set SN" {
            n202 = Unbundle By Name(w390) -> ("Connected"=w389:bool)
            n203 = case shown="True" w389 {
              tunnel: [_ w397] -> w393
              tunnel: w390 -> [_ w396]
              tunnel: w391 -> [_ w395]
              tunnel: "SN Input" -> [_ w394]
              frame False {
              }
              frame True {
                n204 = case shown="False" w395 {
                  tunnel: [w400 _] -> w397
                  tunnel: w396 -> [w403 _]
                  tunnel: w394 -> [w399 w409]
                  frame False {
                    n205 = Unbundle By Name(w403) -> ("Var URLs"=w402:T5[])
                    n206 = for {
                      tunnel: w402 -> [w408] mode=indexing
                      tunnel: [w404] -> w401
                      stop <- w405 stop-if-true
                      n207 = Unbundle By Name(w408) -> ("URL"=w404:string, "Var"=w407:T6)
                      n208 = Equal?(x=w407, y=PLC.Dial800.VarNameSelector."SN" ("Var")) -> (x = y?=w405:bool)
                    }
                    n209 = DataSocket Write(9:100 ("ms timeout (0)"), 10:w399, 11:w401) -> (0:w400:errorcluster)  [unwired: 1 in, 2 out]
                  }
                  frame True {
                    n210 = local read "PLC Variables"() -> (w411:T2)
                    n211 = Bundle By Name(cluster=w411, "SN"=w409) -> (w412:T2)
                    n212 = Wait (ms)(milliseconds to wait=u32 100) -> ()  [unwired: 1 out]
                    n213 = local write "PLC Variables"(w412) -> ()
                  }
                }
              }
            }
            n214 = local write "Status"("Set SN" ("Activity")) -> ()
          }
          frame "PLC - Set Result" {
            n215 = local read "Result"() -> (w417:string)
            n216 = Unbundle By Name(w419) -> ("Connected"=w418:bool)
            n217 = Equal?(x=w417, y="PASS") -> (x = y?=w421:bool)
            n218 = Empty String/Path?(string/path=w417) -> (empty?=w413:bool)
            n219 = case shown="True" w418 {
              tunnel: [_ w427] -> w423
              tunnel: w421 -> [_ w426]
              tunnel: w419 -> [_ w425]
              tunnel: w420 -> [_ w424]
              frame False {
              }
              frame True {
                n220 = case shown="False" w424 {
                  tunnel: [w429 _] -> w427
                  tunnel: w426 -> [w428 w439]
                  tunnel: w425 -> [w430 _]
                  frame False {
                    n221 = Unbundle By Name(w430) -> ("Var URLs"=w433:T5[])
                    n222 = for {
                      tunnel: w433 -> [w438] mode=indexing
                      tunnel: [w434] -> w432
                      stop <- w435 stop-if-true
                      n223 = Unbundle By Name(w438) -> ("URL"=w434:string, "Var"=w437:T6)
                      n224 = Equal?(x=w437, y=PLC.Dial800.VarNameSelector."Pass" ("Var")) -> (x = y?=w435:bool)
                    }
                    n225 = DataSocket Write(9:100 ("ms timeout (0)"), 10:w428, 11:w432) -> (0:w429:errorcluster)  [unwired: 1 in, 2 out]
                  }
                  frame True {
                    n226 = local read "PLC Variables"() -> (w440:T2)
                    n227 = Bundle By Name(cluster=w440, "Pass"=w439) -> (w441:T2)
                    n228 = Wait (ms)(milliseconds to wait=u32 100) -> ()  [unwired: 1 out]
                    n229 = local write "PLC Variables"(w441) -> ()
                  }
                }
              }
            }
            n230 = Select(t="Cleared Result" ("Activity"), s=w413, f="Set Result" ("Activity")) -> (s? t:f=w414:string)
            n231 = local write "Status"(w414) -> ()
          }
          frame "HeartBeat - Test PC" {
            n232 = Unbundle By Name(w446) -> ("Connected"=w452:bool)
            n233 = Unbundle By Name(w446) -> ("HeartBeat"=w450:bool)
            n234 = case shown="True" w452 {
              tunnel: [_ w457] -> w451
              tunnel: w446 -> [_ w456]
              tunnel: w453 -> [_ w455]
              tunnel: w450 -> [_ w454]
              frame False {
              }
              frame True {
                n235 = case shown="True" w455 {
                  tunnel: [w460 _] -> w457
                  tunnel: w456 -> [w463 _]
                  tunnel: w454 -> [w459 w469]
                  frame False {
                    n236 = Unbundle By Name(w463) -> ("Var URLs"=w462:T5[])
                    n237 = for {
                      tunnel: w462 -> [w468] mode=indexing
                      tunnel: [w464] -> w461
                      stop <- w465 stop-if-true
                      n238 = Unbundle By Name(w468) -> ("URL"=w464:string, "Var"=w467:T6)
                      n239 = Equal?(x=w467, y=PLC.Dial800.VarNameSelector."Heartbeat_PC" ("Var")) -> (x = y?=w465:bool)
                    }
                    n240 = DataSocket Write(9:100 ("ms timeout (0)"), 10:w459, 11:w461) -> (0:w460:errorcluster)  [unwired: 1 in, 2 out]
                  }
                  frame True {
                    n241 = local read "PLC Variables"() -> (w471:T2)
                    n242 = Bundle By Name(cluster=w471, "Heartbeat TestPC"=w469) -> (w472:T2)
                    n243 = Wait (ms)(milliseconds to wait=u32 100) -> ()  [unwired: 1 out]
                    n244 = local write "PLC Variables"(w472) -> ()
                  }
                }
              }
            }
            n245 = Unbundle By Name(w446) -> ("HeartBeat"=w447:bool)
            n246 = Not(x=w447) -> (.not. x?=w448:bool)
            n247 = Bundle By Name(cluster=w446, "HeartBeat"=w448) -> (w449:T11)
            n248 = call <vilib>:"Q.Enqueue Task.vi"("Top of Q"=TRUE, "Task Name"="HeartBeat Ck - PLC", "Q In"=w443) -> ()  [unwired: 7 in, 2 out]
          }
          frame "HeartBeat Ck - PLC" {
            n249 = Unbundle By Name(w479) -> ("HB PLC Trans"=w475:timestamp, "HB PLC Last State"=w477:bool)
            n250 = local read "PLC Variables"() -> (w480:T2)
            n251 = Unbundle By Name(w480) -> ("Heartbeat PLC"=w476:bool)
            n252 = Not Equal?(x=w477, y=w476) -> (x != y?=w474:bool)
            n253 = case shown="False" w474 {
              tunnel: w476 -> [_ w497]
              tunnel: w479 -> [w482 w498]
              tunnel: [w483 w496] -> w478
              tunnel: w475 -> [w488 _]
              tunnel: w473 -> [w484 _]
              frame False {
                n254 = Get Date/Time In Seconds() -> (seconds since 1Jan1904=w489:timestamp)
                n255 = Subtract(x=w489, y=w488) -> (x-y=w487:dbl)
                n256 = Greater?(x=w487, y="PLC HB TimeOut(s)") -> (0:w485:bool)
                n257 = case shown="True" w485 {
                  tunnel: w484 -> [_ w493]
                  tunnel: [_ TRUE] -> w481
                  frame False {
                  }
                  frame True {
                    n258 = call <vilib>:"Q.Enqueue Task.vi"("Top of Q"=TRUE, "Task Name"="Reset Due to HB or Cmd", "Q In"=w493) -> ()  [unwired: 7 in, 2 out]
                  }
                }
                n259 = Bundle By Name(cluster=w482, "PLC HB Err"=w481) -> (w483:T11)
                n260 = property on="PLC HB Err Msg" class="Str"("Visible"=w481) -> ()  [unwired: 2 in, 2 out]
                n261 = local write "PLC HB Err"(w481) -> ()
              }
              frame True {
                n262 = Get Date/Time In Seconds() -> (seconds since 1Jan1904=w495:timestamp)
                n263 = Bundle By Name(cluster=w498, "PLC HB Err"=FALSE, "HB PLC Last State"=w497, "HB PLC Trans"=w495) -> (w496:T11)
              }
            }
          }
          frame "Reset Due to HB or Cmd" {
            n264 = Unbundle By Name(w500) -> ("State"=w501:T1)
            n265 = case shown="Default" w501 {
              tunnel: w503 -> [_ w515]
              tunnel: w502 -> [_ w514]
              tunnel: w500 -> [w504 w507]
              tunnel: [w504 w505] -> w499
              frame "Idle" {
                # "Do Nothing"
              }
              frame Default {
                n266 = Not A Number/Path/Refnum?(number/path/refnum=w515) -> (NaN/Path/Refnum?=w522:bool)
                n267 = local write "Result"("" ("Result")) -> ()
                n268 = To Variant(anything=FALSE ("Top of Q")) -> (Variant=w509:variant)
                n269 = case shown="False" w522 {
                  tunnel: w515 -> [w526 _]
                  tunnel: "Test Abort" -> [w525 _]
                  frame False {
                    n270 = call <vilib>:"Q.Enqueue Seq.vi"("Seq Task Name"=w525, "Q In"=w526) -> ()  [unwired: 8 in, 2 out]
                  }
                  frame True {
                  }
                }
                n271 = call <vilib>:"Q.Enqueue Task.vi"("Data1"=w509, "Task Name"="PLC - Set Running", "Q In"=w514) -> ("Q Out"=w524:refnum<queue>)  [unwired: 7 in, 1 out]
                n272 = call <vilib>:"Q.Enqueue Task.vi"("Data1"=w509, "Task Name"="PLC - Set Done", "Q In"=w524) -> ("Q Out"=w523:refnum<queue>)  [unwired: 7 in, 1 out]
                n273 = call <vilib>:"Q.Enqueue Task.vi"("Task Name"="PLC - Set Result", "Q In"=w523) -> ("Q Out"=w511:refnum<queue>)  [unwired: 8 in, 1 out]
                n274 = call <vilib>:"Q.Enqueue Task.vi"("Data1"=w509, "Task Name"="PLC - Set Start", "Q In"=w511) -> ("Q Out"=w510:refnum<queue>)  [unwired: 7 in, 1 out]
                n275 = Bundle By Name(cluster=w507, "State"=T1."Idle") -> (w505:T11)
                n276 = call <vilib>:"Q.Enqueue Reset.vi"("Top of Q(T)"=FALSE, "Flush Queue(T)"=FALSE, "Q In"=w510) -> ()  [unwired: 7 in, 2 out]
              }
            }
          }
          frame "State Check" {
            n277 = Unbundle By Name(w528) -> ("Data"=w529:T2, "State"=w533:T1)
            n278 = Unbundle By Name(w529) -> ("Reset"=w527:bool)
            n279 = case shown="True" w527 {
              tunnel: w533 -> [w540 _]
              tunnel: w532 -> [w539 w631]
              tunnel: [w538 w626] -> w531
              tunnel: w530 -> [w537 w625]
              tunnel: w528 -> [w536 w627]
              tunnel: w529 -> [w535 _]
              tunnel: w528 -> [w534 w622]
              frame False {
                n280 = case shown="\"Idle\", Default" w540 {
                  tunnel: w535 -> [w551 _ _ _ w606]
                  tunnel: w539 -> [w550 _ w580 w596 w604]
                  tunnel: w536 -> [w549 w579 w587 w602 w608]
                  tunnel: [w548 w578 w586 w601 w607] -> w538
                  tunnel: w537 -> [_ _ _ _ _]
                  tunnel: w534 -> [w545 _ w585 _ _]
                  frame "Idle", Default {
                    n281 = Unbundle By Name(w545) -> ("PLC HB Err"=w544:bool)
                    n282 = Unbundle By Name(w551) -> ("Start"=w546:bool)
                    n283 = Not(x=w544) -> (.not. x?=w541:bool)
                    n284 = And(x="Enabled", y=w546) -> (x .and. y?=w543:bool)
                    n285 = And(x=w543, y=w541) -> (x .and. y?=w542:bool)
                    n286 = case shown="True" w542 {
                      tunnel: w550 -> [_ w571]
                      tunnel: w549 -> [w552 w575]
                      tunnel: [w552 w574] -> w548
                      frame False {
                        # "Do Nothing"
                      }
                      frame True {
                        w573 = T1."Setup" ("Test State")
                        n287 = local write "Result"("" ("Result")) -> ()
                        n288 = Wait (ms)(milliseconds to wait=u32 100) -> ()  [unwired: 1 out]
                        n289 = To Variant(anything=FALSE ("Top of Q")) -> (Variant=w554:variant)
                        n290 = call <vilib>:"Q.Enqueue Task.vi"("Top of Q"=TRUE, "Task Name"="Load SN and Nest", "Q In"=w571) -> ("Q Out"=w563:refnum<queue>)  [unwired: 7 in, 1 out]
                        n291 = To Variant(anything=TRUE ("Top of Q")) -> (Variant=w564:variant)
                        n292 = call <vilib>:"Q.Enqueue Task.vi"("Data1"=w554, "Task Name"="PLC - Set Done", "Q In"=w563) -> ("Q Out"=w558:refnum<queue>)  [unwired: 7 in, 1 out]
                        n293 = call <vilib>:"Q.Enqueue Task.vi"("Task Name"="PLC - Set Result", "Q In"=w558) -> ("Q Out"=w557:refnum<queue>)  [unwired: 8 in, 1 out]
                        n294 = Bundle By Name(cluster=w575, "Reset"=FALSE ("TE Running"), "TE Running"=FALSE, "Cleanup"=FALSE, "State"=w573) -> (w574:T11)
                        n295 = local write "Test State"(w573) -> ()
                        n296 = call <vilib>:"Q.Enqueue Task.vi"("Data1"=w564, "Task Name"="PLC - Set Running", "Q In"=w557) -> ("Q Out"=w567:refnum<queue>)  [unwired: 7 in, 1 out]
                        n297 = call <vilib>:"Q.Enqueue Task.vi"("Task Name"="TE Launch", "Q In"=w567) -> ()  [unwired: 8 in, 2 out]
                      }
                    }
                  }
                  frame "Setup" {
                    w577 = T1."Running" ("Test State")
                    n298 = Wait (ms)(milliseconds to wait=u32 50) -> ()  [unwired: 1 out]
                    n299 = local write "Test State"(w577) -> ()
                    n300 = Bundle By Name(cluster=w579, "State"=w577) -> (w578:T11)
                  }
                  frame "Running" {
                    n301 = Unbundle By Name(w585) -> ("Cleanup"=w583:bool, "TE Running"=w581:bool)
                    n302 = Not(x=w581) -> (.not. x?=w582:bool)
                    n303 = Or(x=w583, y=w582) -> (x .or. y?=w584:bool)
                    n304 = case shown="True" w584 {
                      tunnel: w587 -> [w588 w595]
                      tunnel: [w588 w594] -> w586
                      tunnel: w580 -> [_ w591]
                      frame False {
                      }
                      frame True {
                        w593 = T1."Cleanup" ("Test State")
                        n305 = To Variant(anything=FALSE) -> (Variant=w590:variant)
                        n306 = local write "Test State"(w593) -> ()
                        n307 = Bundle By Name(cluster=w595, "State"=w593) -> (w594:T11)
                        n308 = call <vilib>:"Q.Enqueue Task.vi"("Data1"=w590, "Task Name"="PLC - Set Running", "Q In"=w591) -> ()  [unwired: 7 in, 2 out]
                      }
                    }
                  }
                  frame "Cleanup" {
                    w603 = T1."Completed" ("Test State")
                    n309 = To Variant(anything=TRUE) -> (Variant=w598:variant)
                    n310 = Wait (ms)(milliseconds to wait=u32 50) -> ()  [unwired: 1 out]
                    n311 = call <vilib>:"Q.Enqueue Task.vi"("Data1"=w598, "Task Name"="PLC - Set Done", "Q In"=w596) -> ()  [unwired: 7 in, 2 out]
                    n312 = local write "Test State"(w603) -> ()
                    n313 = Bundle By Name(cluster=w602, "State"=w603) -> (w601:T11)
                  }
                  frame "Completed" {
                    # "Wait for Start to be Cleared"
                    n314 = Unbundle By Name(w606) -> ("Start"=w605:bool)
                    n315 = case shown="False" w605 {
                      tunnel: w608 -> [w619 w620]
                      tunnel: [w618 w620] -> w607
                      tunnel: w604 -> [w609 _]
                      frame False {
                        w617 = T1."Idle" ("Test State")
                        n316 = local write "Result"("" ("Result")) -> ()
                        n317 = To Variant(anything=FALSE ("Top of Q")) -> (Variant=w614:variant)
                        n318 = Wait (ms)(milliseconds to wait=u32 100) -> ()  [unwired: 1 out]
                        n319 = call <vilib>:"Q.Enqueue Task.vi"("Data1"=w614, "Task Name"="PLC - Set Done", "Q In"=w609) -> ("Q Out"=w615:refnum<queue>)  [unwired: 7 in, 1 out]
                        n320 = local write "Test State"(w617) -> ()
                        n321 = Bundle By Name(cluster=w619, "State"=w617) -> (w618:T11)
                        n322 = call <vilib>:"Q.Enqueue Task.vi"("Task Name"="PLC - Set Result", "Q In"=w615) -> ()  [unwired: 8 in, 2 out]
                      }
                      frame True {
                      }
                    }
                  }
                }
              }
              frame True {
                w624 = FALSE ("Blinking")
                w630 = T1."Idle" ("Test State")
                # "Reset Command form PLC"
                n323 = Unbundle By Name(w622) -> ("Reset"=w621:bool)
                n324 = case shown="False" w621 {
                  tunnel: w631 -> [w636 _]
                  tunnel: w625 -> [w634 _]
                  frame False {
                    # "Only send TE Reset and re-init once"
                    n325 = Not A Number/Path/Refnum?(number/path/refnum=w634) -> (NaN/Path/Refnum?=w633:bool)
                    n326 = local write "Result"("" ("Result")) -> ()
                    n327 = To Variant(anything=FALSE ("Top of Q")) -> (Variant=w635:variant)
                    n328 = case shown="False" w633 {
                      tunnel: w634 -> [w645 _]
                      tunnel: "Test Abort" -> [w644 _]
                      frame False {
                        n329 = call <vilib>:"Q.Enqueue Seq.vi"("Seq Task Name"=w644, "Q In"=w645) -> ()  [unwired: 8 in, 2 out]
                      }
                      frame True {
                      }
                    }
                    n330 = call <vilib>:"Q.Enqueue Task.vi"("Data1"=w635, "Task Name"="PLC - Set Running", "Q In"=w636) -> ("Q Out"=w643:refnum<queue>)  [unwired: 7 in, 1 out]
                    n331 = call <vilib>:"Q.Enqueue Task.vi"("Data1"=w635, "Task Name"="PLC - Set Done", "Q In"=w643) -> ("Q Out"=w642:refnum<queue>)  [unwired: 7 in, 1 out]
                    n332 = call <vilib>:"Q.Enqueue Task.vi"("Task Name"="PLC - Set Result", "Q In"=w642) -> ()  [unwired: 8 in, 2 out]
                  }
                  frame True {
                    n333 = Wait (ms)(milliseconds to wait=u32 100) -> ()  [unwired: 1 out]
                  }
                }
                n334 = invoke on="SN" class="Str" method="Reinit To Default"() -> ()  [unwired: 3 in, 3 out]
                n335 = Bundle By Name(cluster=w627, "Reset"=TRUE ("TE Running"), "TE Running"=FALSE, "Cleanup"=FALSE, "State"=w630) -> (w626:T11)
                n336 = local write "Test State"(w630) -> ()
                n337 = property on="Test Running" class="Bool (strict)"("Blinking"=w624, "Value"=w624) -> ()  [unwired: 2 in, 2 out]
              }
            }
          }
          frame "Show Panel" {
            n338 = control-ref of="This VI"() -> (w647:refnum<vi>)
            n339 = invoke class="VI" method="FP.Center"(reference=w647) -> (reference out=w650:refnum<vi>, error out=w651:errorcluster)  [unwired: 2 in, 1 out]
            n340 = invoke class="VI" method="FP.Open"(reference=w650, error in=w651, "Activate"=TRUE ("Activate?"), "State"=T9."Standard") -> ()  [unwired: 1 in, 5 out]
          }
          frame "TE Complete" {
            w661 = FALSE ("Blinking")
            # "Message From TE"
            n341 = property on="Test Running" class="Bool (strict)"("Blinking"=w661, "Value"=w661) -> ()  [unwired: 2 in, 2 out]
            n342 = To Variant(anything=FALSE) -> (Variant=w659:variant)
            n343 = invoke on="SN" class="Str" method="Reinit To Default"() -> ()  [unwired: 3 in, 3 out]
            n344 = call <vilib>:"Q.Enqueue Task.vi"("Data1"=w659, "Task Name"="PLC - Set Running", "Q In"=w660) -> ("Q Out"=w653:refnum<queue>)  [unwired: 7 in, 1 out]
            n345 = Bundle By Name(cluster=w663, "TE Running"=FALSE) -> (w662:T11)
            n346 = To Variant(anything=TRUE) -> (Variant=w655:variant)
            n347 = call <vilib>:"Q.Enqueue Task.vi"("Data1"=w655, "Task Name"="PLC - Set Done", "Q In"=w653) -> ()  [unwired: 7 in, 2 out]
          }
          frame "TE Enable PLC" {
            n348 = Variant To Data(type=FALSE, Variant=w667) -> (data=w665:bool)  [unwired: 1 in, 1 out]
            n349 = local write "Enabled"(w665) -> ()
          }
          frame "TE Idle" {
            # "Message From TE"
          }
          frame "TE PLC Start" {
            n350 = call <vilib>:"Q.Enqueue Task.vi"("Task Name"="PLC - Set Start", "Q In"=w671) -> ()  [unwired: 8 in, 2 out]
          }
          frame "TE Launch" {
            # "Message to TE"
            n351 = case shown="True" w678 {
              tunnel: w679 -> [_ w695]
              tunnel: [_ w692] -> _
              frame False {
              }
              frame True {
                n352 = local read "Nest"() -> (w683:i32)
                n353 = local read "SN"() -> (w684:string)
                n354 = Number To Decimal String(number=w683) -> (decimal integer string=w682:string)  [unwired: 1 in]
                n355 = call <vilib>:"Q.Enqueue Seq.vi"("Seq Task Name"="Test Reset" ("Task Name"), "Q In"=w695) -> ("Q Out"=w686:refnum<queue>)  [unwired: 8 in, 1 out]
                n356 = To Variant(anything=w684) -> (Variant=w691:variant)
                n357 = call <vilib>:"Q.Enqueue Task.vi"("Data1"=w691, "Task Name"="Set SN", "Q In"=w686) -> ("Q Out"=w687:refnum<queue>)  [unwired: 7 in, 1 out]
                n358 = To Variant(anything=w682) -> (Variant=w689:variant)
                n359 = call <vilib>:"Q.Enqueue Task.vi"("Data1"=w689, "Task Name"="Set UUT Pos", "Q In"=w687) -> ("Q Out"=w685:refnum<queue>)  [unwired: 7 in, 1 out]
                n360 = call <vilib>:"Q.Enqueue Seq.vi"("Seq Task Name"="Test Start", "Q In"=w685) -> ("error out"=w692:errorcluster)  [unwired: 8 in, 1 out]
              }
            }
            n361 = case shown="True" w673 {
              tunnel: w674 -> [_ w680]
              frame False {
              }
              frame True {
                n362 = call <vilib>:"Q.Enqueue Task.vi"("Task Name"="TE Running", "Q In"=w680) -> ()  [unwired: 8 in, 2 out]
              }
            }
            n363 = Bundle By Name(cluster=w677, "TE Running"=TRUE) -> (w676:T11)
          }
          frame "TE Result" {
            # "Message From TE"
            n364 = Variant To Data(type="", Variant=w703) -> (data=→"Result":string)  [unwired: 1 in, 1 out]
            n365 = call <vilib>:"Q.Enqueue Task.vi"("Task Name"="PLC - Set Result", "Q In"=w700) -> ()  [unwired: 8 in, 2 out]
            n366 = Bundle By Name(cluster=w698, "Cleanup"=TRUE) -> (w697:T11)
          }
          frame "TE Running" {
            # "Message From TE"
            n367 = To Variant(anything=TRUE ("Top of Q")) -> (Variant=w707:variant)
            n368 = call <vilib>:"Q.Enqueue Task.vi"("Data1"=w707, "Task Name"="PLC - Set Running", "Q In"=w710) -> ()  [unwired: 7 in, 2 out]
            n369 = property on="Test Running" class="Bool (strict)"("Blinking"=TRUE) -> ()  [unwired: 2 in, 2 out]
            n370 = Bundle By Name(cluster=w705, "TE Running"=TRUE) -> (w704:T11)
            "Test Running" <- TRUE ("Test Running")
          }
          frame Default {
          }
        }
      }
      frame "Error", Default {
        n371 = case shown="Default" w719 {
          tunnel: w718 -> [_ w723 _]
          tunnel: [w720 w723 _] -> w717
          tunnel: w716 -> [w722 _ _]
          frame "Error" {
            n372 = Variant To Data(type=errorcluster {"status"=FALSE, "code"=0, "source"=""} ("error constant"), Variant=w722) -> (data=w720:errorcluster)  [unwired: 1 in, 1 out]
          }
          frame Default {
          }
          frame "Clear" {
          }
        }
        "Error" <- w717
        n373 = Get Date/Time In Seconds() -> (seconds since 1Jan1904=→"Error Time":timestamp)
      }
      frame "Exit" {
        # "Changed from read using connection ref to using URL"
        n374 = call <vilib>:"Scheduler.Clear-Reset.vi"("Q In"=w725) -> ()  [unwired: 9 in, 2 out]
        n375 = property class="App"() -> ("App.Kind"=w730:T7)  [unwired: 2 in, 2 out]
        n376 = Generate User Event(user event=w733, event data cluster=TRUE ("event data")) -> ()  [unwired: 2 in, 2 out]
        n377 = Equal?(x=w730, y=T7."Run Time System" ("Application:Kind")) -> (x = y?=w728:bool)
        n378 = case shown="True" w728 {
          frame False {
          }
          frame True {
            n379 = control-ref of="This VI"() -> (w742:refnum<vi>)
            n380 = property class="VI"(reference=w742, "FP.State"=T9."Closed" ("Front Panel Window:State")) -> ()  [unwired: 1 in, 2 out]
          }
        }
        n381 = case shown="False" w731 {
          frame False {
            n382 = call <vilib>:"Scheduler.Exit.vi"() -> ()  [unwired: 11 in, 1 out]
          }
          frame True {
          }
        }
        n383 = disable-structure shown="Disabled" {
          disable-tunnel: w727 -> [w736 _]
          disable-tunnel: w726 -> [w735 _]
          frame Disabled {
            n384 = case shown="False" w736 {
              tunnel: w735 -> [w740 _]
              frame False {
                n385 = Unbundle By Name(w740) -> ("Var URLs"=w739:T5[])
                n386 = call "PLC.Dial800.OPC Disconnect.vi"("ms timeout (1000)"=100, "Var URLs In"=w739) -> ("error out"=w737:errorcluster)  [unwired: 9 in]
                n387 = call <vilib>:"Clear Errors.vi"("error in (no error)"=w737) -> ()  [unwired: 5 in, 2 out]
              }
              frame True {
              }
            }
          }
          frame Enabled {
          }
        }
        n388 = call <vilib>:"Activity Light - Exit.vi"("Name"="Read Light" ("Q Name")) -> ()  [unwired: 10 in, 1 out]
      }
    }
  }
  n389 = control-ref of="Reading"() -> (w1:refnum<vi>)
  n390 = call <vilib>:"Activity Light - Core.vi"("Bool Refnum"=w1, "Q Name"="Read Light") -> ()  [unwired: 1 in]
